vi "Two Asymmetric Gaussians Fit Guess Parameters.vi"(8 "Cursor X 2":dbl, 9 "Cursor X 1":dbl, 10 "Y Array":dbl[](array[numeric]), 11 "X Array":dbl[](array[numeric])) -> (1 "Guess Parameters Array":dbl[](array[numeric]), 2 "Y Array dup":dbl[](array[numeric]), 3 "X Array dup":dbl[](array[numeric]))   [LabVIEW 2021, in "Fits.lvlib"]
uses:
  Fits.lvlib
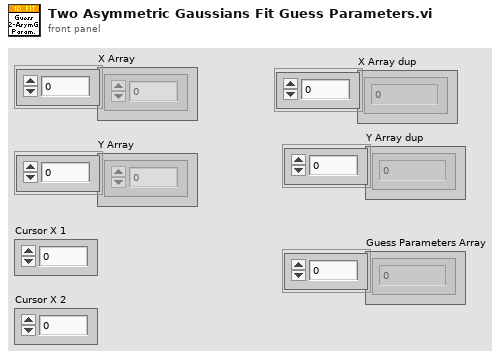
[diagram p1: front panel]
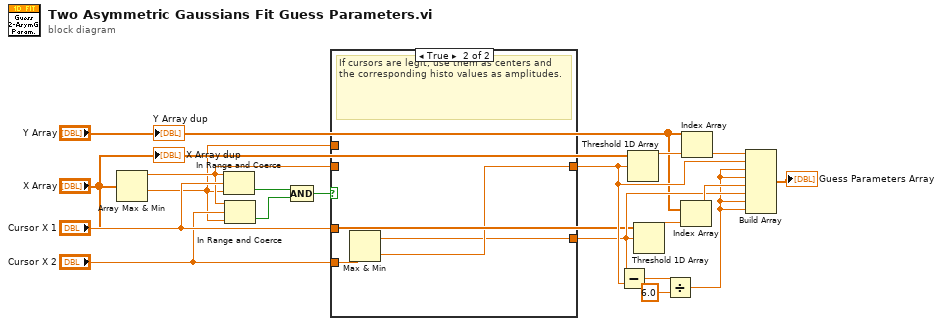
[diagram p0: block diagram]
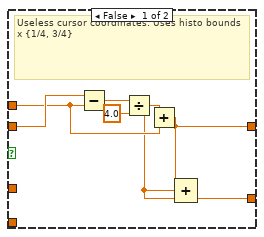
[diagram p2: hidden frame]
diagram:
  n1 = Array Max & Min(array="X Array") -> (max value=w4:dbl, min value=w3:dbl)  [unwired: 2 out]
  n2 = In Range and Coerce(upper limit=w4, x="Cursor X 1", lower limit=w3) -> (In Range?=w19:bool)  [unwired: 1 out]
  n3 = In Range and Coerce(upper limit=w4, x="Cursor X 2", lower limit=w3) -> (In Range?=w18:bool)  [unwired: 1 out]
  n4 = Compound Arithmetic op=AND(w19, w18) -> (w17:bool)
  n5 = case shown="True" w17 {
    tunnel: "Cursor X 1" -> [_ w30]
    tunnel: "Cursor X 2" -> [_ w29]
    tunnel: [w22 w28] -> w8
    tunnel: [w20 w27] -> w7
    tunnel: w4 -> [w24 _]
    tunnel: w3 -> [w23 _]
    frame False {
      # "Useless cursor coordinates. Uses histo bounds x {1/4, 3/4}"
      n6 = Subtract(x=w24, y=w23) -> (x-y=w26:dbl)
      n7 = Divide(x=w26, y=4.0) -> (x/y=w21:dbl)
      n8 = Add(x=w21, y=w23) -> (x+y=w22:dbl)
      n9 = Compound Arithmetic op=ADD(w22, w21, w21) -> (w20:dbl)
    }
    frame True {
      # "If cursors are legit, use them as centers and the corresponding histo values as amplitudes."
      n10 = Max & Min(x=w30, y=w29) -> (max(x,y)=w27:dbl, min(x,y)=w28:dbl)
    }
  }
  n11 = Subtract(x=w7, y=w8) -> (x-y=w11:dbl)
  n12 = Threshold 1D Array(2:w8, 3:"X Array") -> (0:w9:dbl)  [unwired: 1 in]
  n13 = Threshold 1D Array(2:w7, 3:"X Array") -> (0:w10:dbl)  [unwired: 1 in]
  n14 = Divide(x=w11, y=6.0) -> (x/y=w1:dbl)
  n15 = Index Array(array="Y Array", index=w10) -> (element=w14:dbl)
  n16 = Index Array(array="Y Array", index=w9) -> (element=w13:dbl)
  n17 = Build Array(w13, w8, w1, w1, w14, w7, w1, w1) -> (→"Guess Parameters Array":dbl[])
  "X Array dup" <- "X Array"
  "Y Array dup" <- "Y Array"
